vi "deeplabv3_onnx.vi"() -> ()   [LabVIEW 2018]
uses:
  <vilib>/addons/VIRobotics/opencv_yiku/ctls/ColorConversionCodes.ctl
  <vilib>/addons/VIRobotics/opencv_yiku/Mat/Mat_32F/Mat_32F.lvclass
  C:/Program Files/National Instruments/LabVIEW 2018/vi.lib/addons/VIRobotics/opencv_yiku/Mat/Mat/Mat.lvclass
  <vilib>/addons/VIRobotics/opencv_yiku/Mat/Mat_8U/Mat_8U.lvclass
  <vilib>/addons/VIRobotics/opencv_yiku/Mat/Mat/Mat_length.vi
  <vilib>/addons/VIRobotics/onnx/Session/get_outputNames.vi
  <vilib>/addons/VIRobotics/onnx/Session/Get_Result_float.vi
  <vilib>/addons/VIRobotics/opencv_yiku/Mat/Mat/Mat_release.vi
  <vilib>/addons/VIRobotics/opencv_yiku/opencv_yiku.lvlib
  <vilib>/addons/VIRobotics/opencv_yiku/Mat/Mat/Mat.lvclass
  <vilib>/addons/VIRobotics/onnx/Session/Session.lvclass
panel:
  out "outputNames":string[](array[string])
  out "mask":picture
  out "原始图像":picture
  out "合成的图像":picture
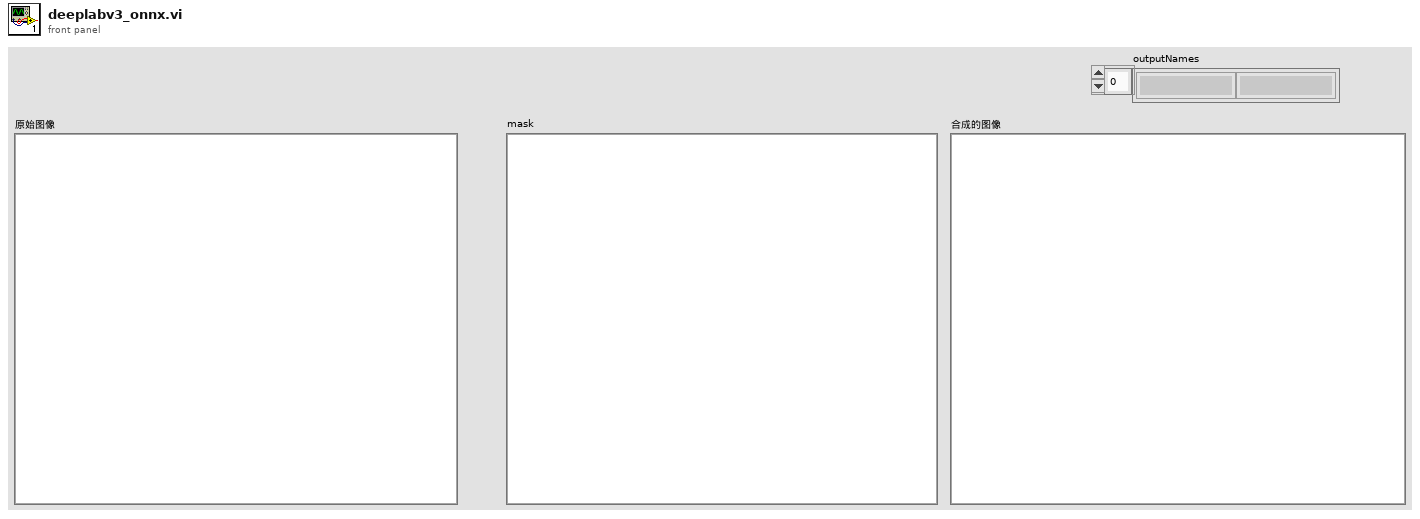
[diagram p1: front panel]
types:
  T1 = typedef "opencv_yiku.lvlib/ColorConversionCodes.ctl" = enum32{"COLOR_BGR2BGRA", "COLOR_BGRA2BGR", "COLOR_BGR2RGBA", "COLOR_RGBA2BGR", "COLOR_BGR2RGB", "COLOR_BGRA2RGBA", "COLOR_BGR2GRAY", "COLOR_RGB2GRAY", "COLOR_GRAY2BGR", "COLOR_GRAY2BGRA", "COLOR_BGRA2GRAY", "COLOR_RGBA2GRAY", "COLOR_BGR2BGR565", "COLOR_RGB2BGR565", "COLOR_BGR5652BGR", "COLOR_BGR5652RGB", "COLOR_BGRA2BGR565", "COLOR_RGBA2BGR565", "COLOR_BGR5652BGRA", "COLOR_BGR5652RGBA", "COLOR_GRAY2BGR565", "COLOR_BGR5652GRAY", "COLOR_BGR2BGR555", "COLOR_RGB2BGR555", "COLOR_BGR5552BGR", "COLOR_BGR5552RGB", "COLOR_BGRA2BGR555", "COLOR_RGBA2BGR555", "COLOR_BGR5552BGRA", "COLOR_BGR5552RGBA", "COLOR_GRAY2BGR555", "COLOR_BGR5552GRAY", "COLOR_BGR2XYZ", "COLOR_RGB2XYZ", "COLOR_XYZ2BGR", "COLOR_XYZ2RGB", "COLOR_BGR2YCrCb", "COLOR_RGB2YCrCb", "COLOR_YCrCb2BGR", "COLOR_YCrCb2RGB", "COLOR_BGR2HSV", "COLOR_RGB2HSV", "42", "43", "COLOR_BGR2Lab", "COLOR_RGB2Lab"}
  T2 = cluster{"height":i32, "width":i32, "channels":i32, "pointer":u64}
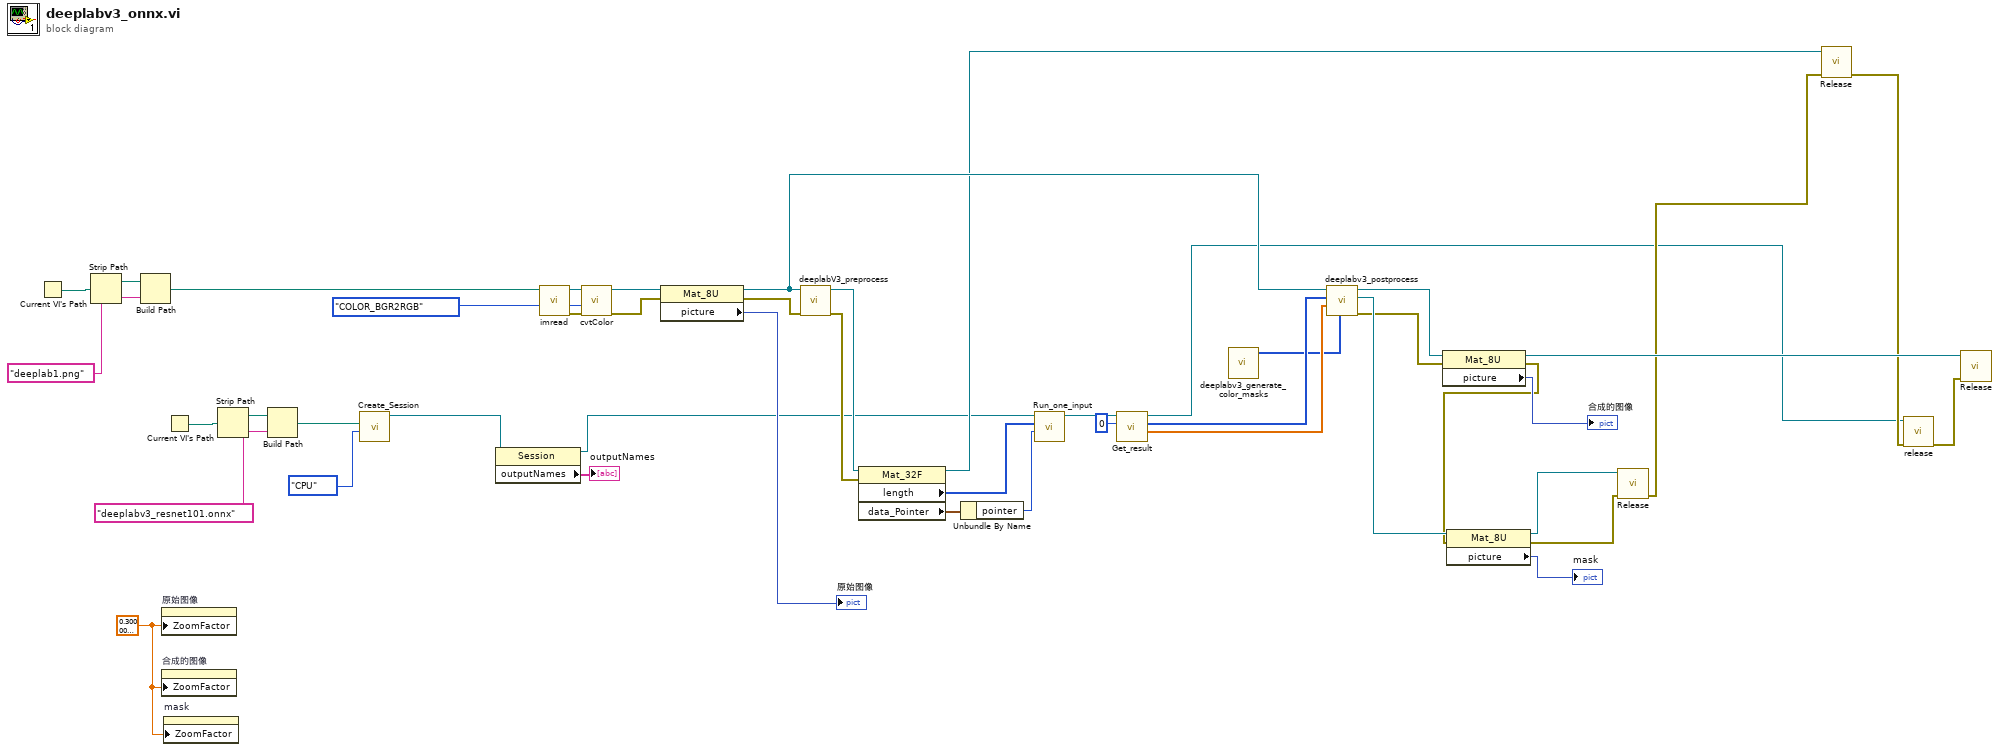
[diagram p0: block diagram]
diagram:
  w25 = sgl 0.3 ("Zoom Factor")
  n1 = Current VI's Path() -> (path=w44:path)
  n2 = Strip Path(path=w44) -> (stripped path=w45:path)  [unwired: 1 out]
  n3 = Build Path(base path=w45, name or relative path="deeplab1.png") -> (appended path=w42:path)
  n4 = property on="原始图像" class="Pict"("ZoomFactor"=w25) -> ()  [unwired: 2 in, 2 out]
  n5 = property on="合成的图像" class="Pict"("ZoomFactor"=w25) -> ()  [unwired: 2 in, 2 out]
  n6 = property on="mask" class="Pict"("ZoomFactor"=w25) -> ()  [unwired: 2 in, 2 out]
  n7 = Current VI's Path() -> (path=w40:path)
  n8 = Strip Path(path=w40) -> (stripped path=w41:path)  [unwired: 1 out]
  n9 = Build Path(base path=w41, name or relative path="deeplabv3_resnet101.onnx") -> (appended path=w19:path)
  n10 = call <vilib>:"Create_Session.vi"("type"=enum16{"CPU", "CUDA", "TensorRT"}."CPU", "path"=w19) -> ("Session out"=w3:refnum<class "Session.lvclass">)  [unwired: 8 in, 1 out]
  n11 = property class="Session"(reference=w3) -> (reference out=w1:refnum<class "Session.lvclass">, "outputNames"=→"outputNames":string[])  [unwired: 1 in, 1 out]
  n12 = call <vilib>:"imread.vi"("path"=w42) -> ("error out"=w36:errorcluster, "Mat out"=w38:refnum<class "Mat_8U.lvclass">)  [unwired: 9 in]
  n13 = call <vilib>:"cvtColor.vi"("error in (no error)"=w36, "dstCn"=ColorConversionCodes."COLOR_BGR2RGB", "src"=w38) -> ("error out"=w29:errorcluster, "src out"=w35:refnum<class "Mat_8U.lvclass">)  [unwired: 6 in, 1 out]
  n14 = property class="Mat_8U"(reference=w35, error in=w29) -> (reference out=w28:refnum<class "Mat_8U.lvclass">, error out=w30:errorcluster, "picture"=→"原始图像":picture)
  n15 = call "deeplabV3_preprocess.vi"("error in (no error)"=w30, "img"=w28) -> ("error out"=w18:errorcluster, "blob"=w17:refnum<class "Mat_32F.lvclass">)  [unwired: 8 in]
  n16 = property class="Mat_32F"(reference=w17, error in=w18) -> (reference out=w6:refnum<class "Mat_32F.lvclass">, "length"=w16:i32[], "data_Pointer"=w15:T2)  [unwired: 1 out]
  n17 = Unbundle By Name(w15) -> ("pointer"=w14:u64)
  n18 = call <vilib>:"Run_one_input.vi"("data_pointer"=w14, "shape"=w16, "Session in"=w1) -> ("Session out"=w13:refnum<class "Session.lvclass">)  [unwired: 6 in, 2 out]
  n19 = call-poly <vilib>:"Get_result.vi"("index"=0, "Session in"=w13) -> ("data"=w10:sgl[], "shape"=w11:i64[], "Session out"=w5:refnum<class "Session.lvclass">)  [unwired: 6 in, 1 out]
  n20 = call "deeplabv3_generate_color_masks.vi"() -> ("colors"=w4:u32[])  [unwired: 11 in]
  n21 = call "deeplabv3_postprocess.vi"("colors"=w4, "1d_data"=w10, "length"=w11, "img in"=w28) -> ("error out"=w23:errorcluster, "mask"=w27:refnum<class "Mat_8U.lvclass">, "img out"=w33:refnum<class "Mat_8U.lvclass">)  [unwired: 5 in]
  n22 = property class="Mat_8U"(reference=w33, error in=w23) -> (reference out=w31:refnum<class "Mat_8U.lvclass">, error out=w21:errorcluster, "picture"=→"合成的图像":picture)
  n23 = property class="Mat_8U"(reference=w27, error in=w21) -> (reference out=w24:refnum<class "Mat_8U.lvclass">, error out=w22:errorcluster, "picture"=→"mask":picture)
  n24 = call-poly <vilib>:"Release.vi"("error in (no error)"=w22, "Mat in"=w24) -> ("error out"=w7:errorcluster)  [unwired: 9 in]
  n25 = call-poly <vilib>:"Release.vi"("error in (no error)"=w7, "Mat in"=w6) -> ("error out"=w9:errorcluster)  [unwired: 9 in]
  n26 = call <vilib>:"release.vi"("error in (no error)"=w9, "Session in"=w5) -> ("error out"=w8:errorcluster)  [unwired: 9 in]
  n27 = call-poly <vilib>:"Release.vi"("error in (no error)"=w8, "Mat in"=w31) -> ()  [unwired: 9 in, 1 out]
